vi "Append Error Description.vi"(0 "error to append":errorcluster, 5 "append string (\"\")":string, 7 "generate error?":bool=TRUE, 11 "error in":errorcluster) -> (15 "error out":errorcluster)   [LabVIEW 2014, in "niHighSpeedSerial Eye Scan Common v1 Host.lvlib"]
doc: "If <b>generate error?</b> is true, this VI sets the specified error on the error chain with the appended error description information.\n\n<B>Input Parameters</B>\n\n<B>error to append</B> 'error to append' is the error code and description which will be set on the 'error out' wire, if 'error in' is not an error.\n\n<B>error to append.status</B> 'status' is TRUE (X) if an error occurred or FALSE (checkmark) to indicate a warning or that no error occurred.\n\nRight-click the 'error in' control on the front panel and select 'Explain Error' or 'Explain Warning' from the shortcut menu for more information about the error.\n\n<B>error to append.code</B> 'code' is the error or warning code.\n\nRight-click the 'error in' control on the front panel and select 'Explain Error' or 'Explain Warning' from the shortcut menu for more information about the error.\n\n<B>error to append.source</B> 'source' describes the origin of the error or warning.\n\nRight-click the 'error in' control on the front panel and select 'Explain Error' or 'Explain Warning' from the shortcut menu for more information about the error.\n\n<B>append string (\"\")</B> Used to provide additional relevant information to the new error value.\n\n<B>generate error?</B> If 'true', causes 'error to append' to be merged into the 'error in' in 'error out'.\n\n<B>error in</B> describes error conditions that occur before this node runs. This input provides standard 'error in' functionality.\n\n<B>Output Parameters</B>\n\n<B>error out</B> contains error information. This output provides standard 'error out' functionality."
uses:
  <instrlib>/niHighSpeedSerial/Eye Scan/v1/Host/Common/niHighSpeedSerial Eye Scan Common v1 Host.lvlib
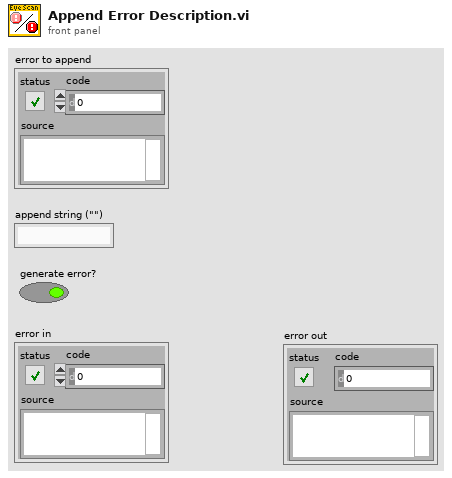
[diagram p1: front panel]
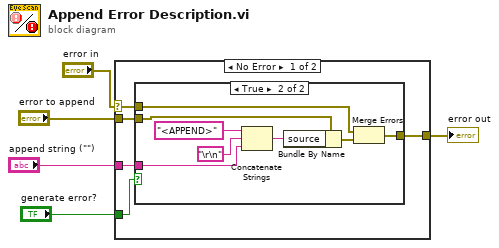
[diagram p0: block diagram]
diagram:
  n1 = case shown="No Error" "error in" {
    selector: "error in" -> [w8 w20]
    tunnel: [w7 w20] -> w4
    tunnel: "generate error?" -> [w6 _]
    tunnel: "error to append" -> [w9 _]
    tunnel: "append string (\"\")" -> [w10 _]
    frame No Error {
      n2 = case shown="True" w6 {
        tunnel: w10 -> [_ w17]
        tunnel: w9 -> [_ w15]
        tunnel: w8 -> [w11 w14]
        tunnel: [w11 w12] -> w7
        frame False {
        }
        frame True {
          n3 = Concatenate Strings("<APPEND>" ("string"), "\r\n", w17) -> (w18:string)
          n4 = Bundle By Name(cluster=w15, "source"=w18) -> (w13:errorcluster)
          n5 = Merge Errors(w14, w13) -> (w12:errorcluster)
        }
      }
    }
    frame Error {
    }
  }
  "error out" <- w4
